vi "Read Reader.vi"(8 "error in (no error)":errorcluster, 11 "ADOResult in":refnum<class "ADOResult.lvclass">) -> (0 "error out":errorcluster, 2 "Reader":refnum<k24>, 3 "ADOResult out":refnum<class "ADOResult.lvclass">)   [LabVIEW 2020, in "ORM_ADONet.lvlib" / "ADOResult.lvclass"]
uses:
  ADOResult.lvclass
  System.Data
  ADOResult.lvclass/ADOResult.ctl
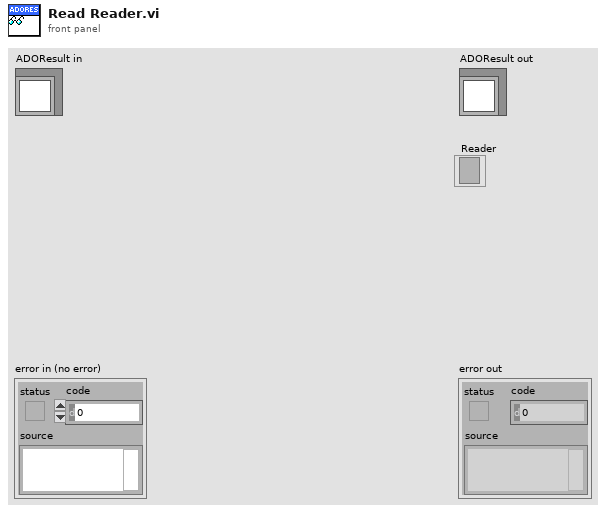
[diagram p1: front panel]
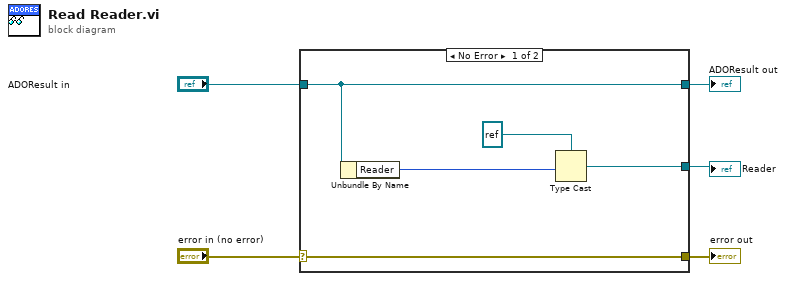
[diagram p0: block diagram]
diagram:
  n1 = case shown="No Error" "error in (no error)" {
    selector: "error in (no error)" -> [w10 w11]
    tunnel: [w10 w11] -> w4
    tunnel: [w9 w12] -> w2
    tunnel: "ADOResult in" -> [w9 w12]
    tunnel: [w6 _] -> w1
    frame No Error {
      n2 = Unbundle By Name(w9) -> ("Reader"=w8:u64)
      n3 = Type Cast(type=refnum<k24> refnum ("Reader"), x=w8) -> (*(type *) &x=w6:refnum<k24>)
    }
    frame Error {
    }
  }
  "error out" <- w4
  "ADOResult out" <- w2
  "Reader" <- w1
